vi "CameraGetKineticSeries.vi"(3 "error out 2":errorcluster, 4 "# of kinetics":i32, 5 "image size":cluster{"xpixels":i32, "ypixels":i32}) -> (0 "error out":errorcluster, 2 "kinetic series data":i32[][][](array[numeric]))   [LabVIEW 2019]
panel:
  out "validlast":i32
  out "validfirst":i32
  out "DLL error code 2":u32
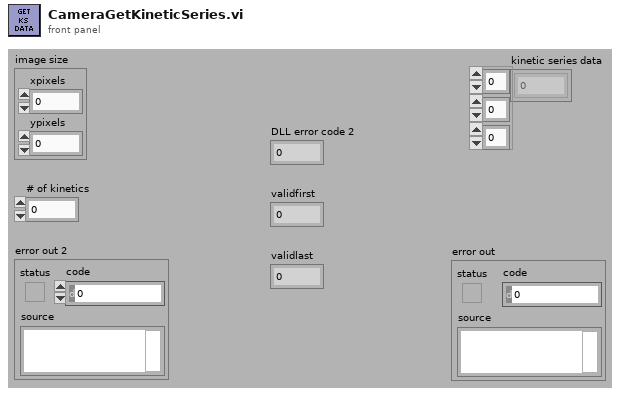
[diagram p1: front panel]
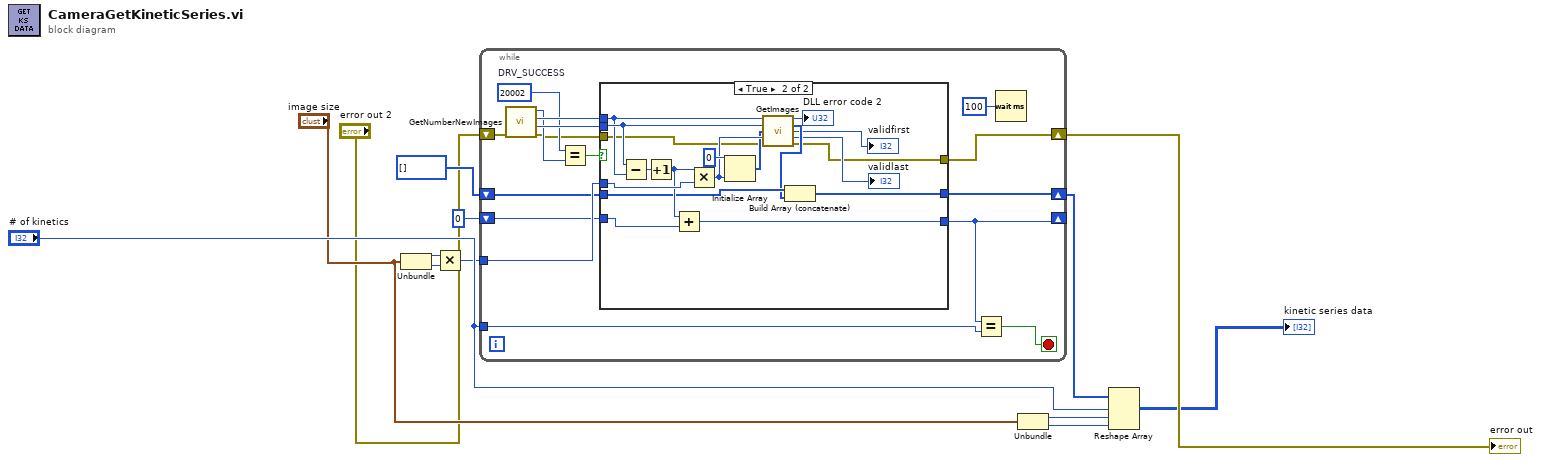
[diagram p0: block diagram]
diagram:
  n1 = Unbundle("image size") -> ("xpixels"=w1:i32, "ypixels"=w2:i32)
  n2 = Multiply(x=w1, y=w2) -> (x*y=w4:i32)
  n3 = while {
    tunnel: w4 -> [w25]
    shift-right: [w21] -> _
    shift-left: 0 -> [w24]
    shift-right: [w22] -> w8
    shift-left: i32[] [] -> [w23]
    tunnel: "# of kinetics" -> [w20]
    shift-right: [w14] -> w13
    shift-left: "error out 2" -> [w29]
    stop <- w19 stop-if-true
    w16 = 20002  # DRV_SUCCESS
    n4 = call <userlib>:"GetNumberNewImages.vi"("error in (no error)"=w29) -> ("error out"=w15:errorcluster, "last"=w26:i32, "first"=w27:u32, "DLL error code"=w17:u32)  [unwired: 3 in]
    n5 = Equal?(x=w16, y=w17) -> (x = y?=w28:bool)
    n6 = case shown="True" w28 {
      tunnel: w27 -> [_ w49]
      tunnel: w26 -> [_ w50]
      tunnel: w25 -> [_ w47]
      tunnel: w24 -> [w32 w44]
      tunnel: [w32 w42] -> w21
      tunnel: w23 -> [w31 w41]
      tunnel: [w31 w39] -> w22
      tunnel: w15 -> [w30 w34]
      tunnel: [w30 w33] -> w14
      frame False {
      }
      frame True {
        n7 = Subtract(x=w50, y=w49) -> (x-y=w48:u32)
        n8 = Increment(x=w48) -> (x+1=w43:u32)
        n9 = Add(x=w43, y=w44) -> (x+y=w42:u32)
        n10 = Multiply(x=w43, y=w47) -> (x*y=w45:u32)
        n11 = Initialize Array(0 ("element"), w45) -> (w40:i32[])
        n12 = call <userlib>:"GetImages.vi"("first"=w49, "last"=w50, "array"=w40, "size"=w45, "error in (no error)"=w34) -> ("DLL error code"=→"DLL error code 2":u32, "array"=w38:i32[], "validfirst"=→"validfirst":i32, "validlast"=→"validlast":i32, "error out"=w33:errorcluster)  [unwired: 6 in]
        n13 = Build Array (concatenate)(w41, w38) -> (w39:i32[])
      }
    }
    n14 = Equal?(x=w21, y=w20) -> (x = y?=w19:bool)
    n15 = Wait (ms)(milliseconds to wait=u32 100) -> ()  [unwired: 1 out]
  }
  "error out" <- w13
  n16 = Unbundle("image size") -> ("xpixels"=w10:i32, "ypixels"=w11:i32)
  n17 = Reshape Array(w8, "# of kinetics", w10, w11) -> (→"kinetic series data":i32[][][])
